vi "Pack Step Value.vi"(8 "error in":errorcluster, 10 "Value":string, 11 "Speaker Step in":refnum<class "Speaker Step.lvclass">) -> (0 "error out":errorcluster, 3 "Speaker Step out":refnum<class "Speaker Step.lvclass">)   [LabVIEW 2017, in "Controller.lvlib" / "Speaker Step.lvclass"]
uses:
  Speaker Step.lvclass
  C:/Program Files (x86)/National Instruments/LabVIEW 2017/vi.lib/MSR Consulting, LLC/General Reuse/Sequence/STEPS/LEAVES/Switch/Switch Step.lvclass
  Speaker Step.lvclass/Speaker Step.ctl
  Write cell.vi
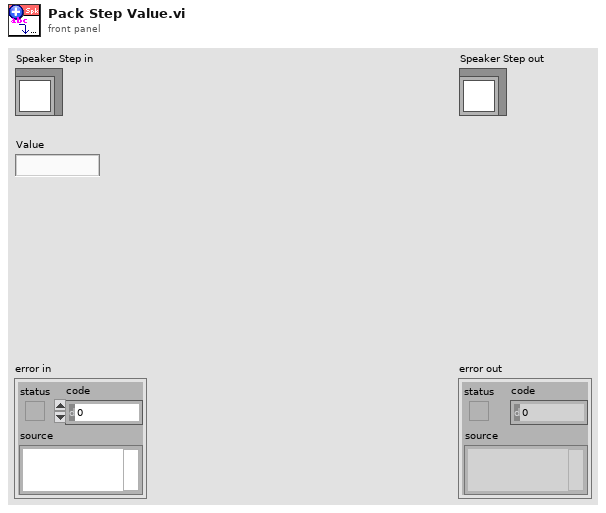
[diagram p1: front panel]
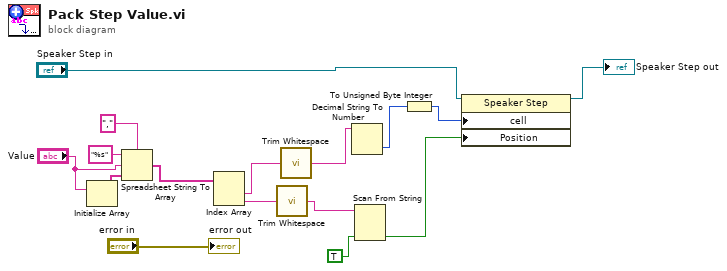
[diagram p0: block diagram]
diagram:
  n1 = Initialize Array("Value") -> (w12:string[])  [unwired: 1 in]
  n2 = Spreadsheet String To Array(delimiter (Tab)=",", format string="%s", spreadsheet string="Value", array type (2D Dbl)=w12) -> (array=w11:string[])
  n3 = Index Array(array=w11) -> (element #1=w10:string, element #2=w9:string)  [unwired: 2 in]
  n4 = call <vilib>:"Trim Whitespace.vi"("string"=w9) -> ("trimmed string"=w7:string)  [unwired: 1 in]
  n5 = call <vilib>:"Trim Whitespace.vi"("string"=w10) -> ("trimmed string"=w8:string)  [unwired: 1 in]
  n6 = Decimal String To Number(string=w8) -> (number=w2:i32)  [unwired: 2 in, 1 out]
  n7 = Scan From String(input string=w7, default 1=TRUE) -> (output 1=w3:bool)  [unwired: 3 in, 3 out]
  n8 = To Unsigned Byte Integer(number=w2) -> (unsigned 8bit integer=w1:u8)
  n9 = property class="Speaker Step"(reference="Speaker Step in", "cell"=w1, "Position"=w3) -> (reference out=→"Speaker Step out":refnum<class "Speaker Step.lvclass">)  [unwired: 1 in, 1 out]
  "error out" <- "error in"
